vi "H5Fget_filesize.vi"(6 "error in (no error)":errorcluster, 9 "HDF5 Ref":T1) -> (0 "error out":errorcluster, 2 "File size":u32, 3 "HDF5 Ref out":T1)   [LabVIEW 2017]
doc: "Returns the size of an HDF5 file.\n\n<p />"
uses:
  <vilib>/UPVI/lvhdf5/library.llb/HDF5 Ref.ctl
  <vilib>/UPVI/lvhdf5/common.llb/U64 to U32.vi
  <vilib>/UPVI/lvhdf5/hdf5.dll
panel:
  # "LVHDF5 Toolkit\nCopyright (c) 2005-2013 by Jason D. Sommerville\nCopyright (c) 2014 by UPVI, LLC.\n\nThis use and distribution of this file is governed by the terms found in \nLICENSE.txt distributed with this toolkit and installed at\n <user.lib>\\_lvhdf5\\LICENSE.txt"
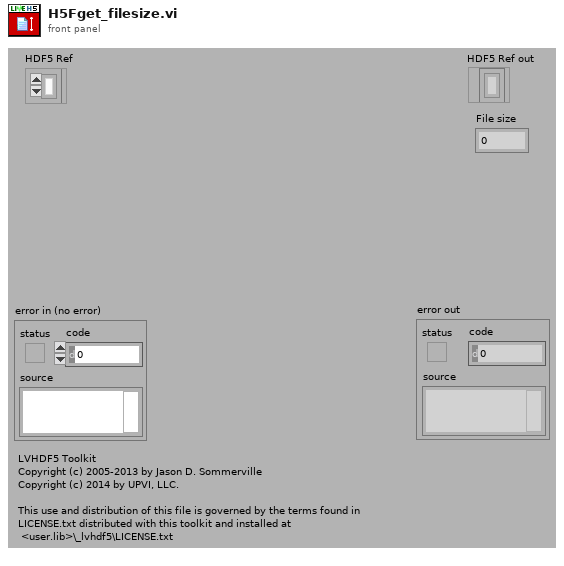
[diagram p1: front panel]
types:
  T1 = typedef "HDF5 Ref.ctl" = refnum<k1>
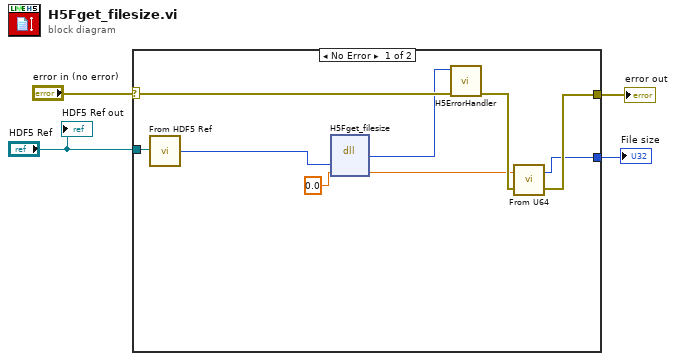
[diagram p0: block diagram]
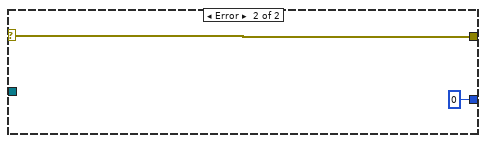
[diagram p2: hidden frame]
diagram:
  n1 = case shown="No Error" "error in (no error)" {
    selector: "error in (no error)" -> [w13 w15]
    tunnel: [w7 w15] -> w3
    tunnel: [w5 u32 0 ("U32")] -> w2
    tunnel: "HDF5 Ref" -> [w10 _]
    frame No Error {
      n2 = call <vilib>:"From HDF5 Ref.vi"("HDF5 Ref"=w10) -> ("I32"=w9:i32)
      n3 = dll-call lib="C:/Program Files/National Instruments/LabVIEW 2017/vi.lib/UPVI/lvhdf5/hdf5.dll" fn="H5Fget_filesize"("file_id"=w9, 0.0 ("input param")) -> (w12:i32, w6:dbl)  [unwired: 4 in, 2 out]
      n4 = call <vilib>:"H5ErrorHandler.vi"("error in (no error)"=w13, "herr_t"=w12) -> ("error out"=w8:errorcluster)  [unwired: 3 in, 4 out]
      n5 = call-poly <vilib>:"From U64.vi"("error in (no error)"=w8, "U64"=w6) -> ("error out"=w7:errorcluster, "U32"=w5:u32)
    }
    frame Error {
    }
  }
  "error out" <- w3
  "File size" <- w2
  "HDF5 Ref out" <- "HDF5 Ref"
